vi "Init.vi"(8 "error in (no error)":errorcluster, 10 "Params":variant, 11 "PIPXI40 Base in":refnum<class "PIPXI40 Base.lvclass">) -> (0 "error out":errorcluster, 3 "PIPXI40 Base out":refnum<class "PIPXI40 Base.lvclass">)   [LabVIEW 2020, in "PIPXI40.lvlib" / "PIPXI40 Base.lvclass"]
uses:
  PIPXI40 Base.lvclass
  PIPXI40 Base.lvclass/PIPXI40 Base.ctl
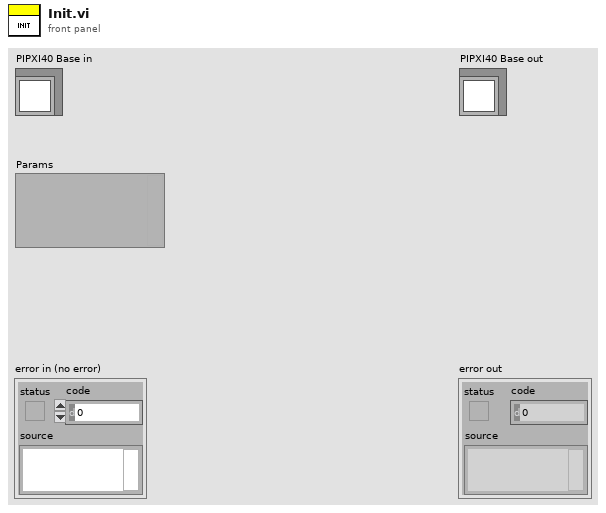
[diagram p1: front panel]
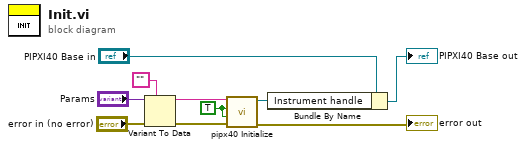
[diagram p0: block diagram]
diagram:
  w6 = TRUE ("reset device")
  n1 = Variant To Data(error in="error in (no error)", type="", Variant="Params") -> (data=w2:string, error out=w4:errorcluster)
  n2 = call <instrlib>:"pipx40 Initialize.vi"("error in (no error)"=w4, "reset device"=w6, "id query"=w6, "resource name"=w2) -> ("error out"=→"error out":errorcluster, "instrument handle out"=w9:refnum<visa-resource-name>)  [unwired: 6 in]
  n3 = Bundle By Name(cluster="PIPXI40 Base in", "Instrument handle"=w9) -> (→"PIPXI40 Base out":refnum<class "PIPXI40 Base.lvclass">)
